vi "GetControlRefnumsOfTab__slk_mt.vi"(8 "error in (no error)":errorcluster, 11 "tab control refnum in":refnum<vi>) -> (0 "error out":errorcluster, 3 "control refnums out":refnum<vi>[](array[refnum]))   [LabVIEW 2010, in "Lazyboots Menu Tool.lvlib"]
doc: "Gets all control refnums from specified tab control."
uses:
  Library/Lazyboots Menu Tool.lvlib
panel:
  # "GetControlRefnumsOfTab__slk_mt.vi\nGets all control refnums from specified tab control.\n\nNOTICE -- YOU MUST LEAVE THIS NOTICE IN PLACE.\n\nCopyright (c) 2011, LIANG LIU Shawn.Liu.cn@gmail.com\nAll rights reserved.\n\nRedistribution and use in source and binary forms, with or without modification, are permitted provided that the following conditions are met:\n-Redistributions of source code must retain the above copyright notice, this list of conditions and the following disclaimer.\n-Redistributions in binary form must reproduce the above copyright notice, this list of conditions and the following disclaimer in the documentation and/or other materials provided with the distribution.\n-Neither the name of the eLp nor the names of its contributors may be used to endorse or promote products derived from this software without specific prior written permission.\n\nTHIS SOFTWARE IS PROVIDED BY THE COPYRIGHT HOLDERS AND CONTRIBUTORS \"AS IS\" AND ANY EXPRESS OR IMPLIED WARRANTIES, INCLUDING, BUT NOT LIMITED TO, THE IMPLIED WARRANTIES OF MERCHANTABILITY AND FITNESS FOR A PARTICULAR PURPOSE ARE DISCLAIMED. IN NO EVENT SHALL THE COPYRIGHT HOLDER OR CONTRIBUTORS BE LIABLE FOR ANY DIRECT, INDIRECT, INCIDENTAL, SPECIAL, EXEMPLARY, OR CONSEQUENTIAL DAMAGES (INCLUDING, BUT NOT LIMITED TO, PROCUREMENT OF SUBSTITUTE GOODS OR SERVICES; LOSS OF USE, DATA, OR PROFITS; OR BUSINESS INTERRUPTION) HOWEVER CAUSED AND ON ANY THEORY OF LIABILITY, WHETHER IN CONTRACT, STRICT LIABILITY, OR TORT (INCLUDING NEGLIGENCE OR OTHERWISE) ARISING IN ANY WAY OUT OF THE USE OF THIS SOFTWARE, EVEN IF ADVISED OF THE POSSIBILITY OF SUCH DAMAGE."
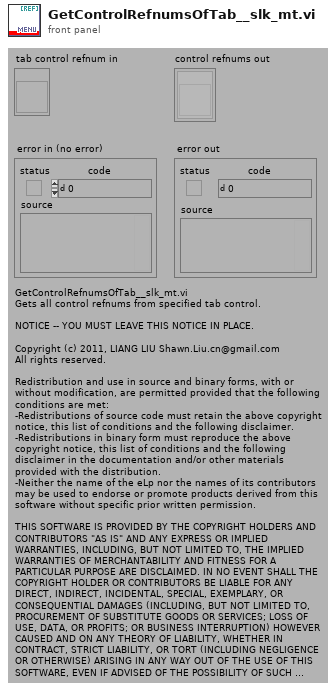
[diagram p1: front panel]
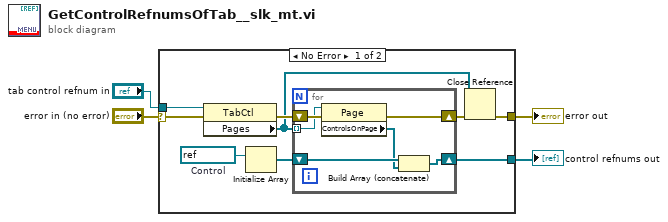
[diagram p0: block diagram]
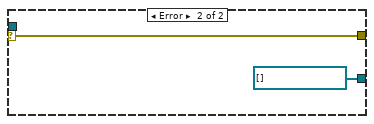
[diagram p2: hidden frame]
diagram:
  n1 = case shown="No Error" "error in (no error)" {
    selector: "error in (no error)" -> [w11 w21]
    tunnel: "tab control refnum in" -> [w13 _]
    tunnel: [w12 refnum<vi>[] []] -> w3
    tunnel: [w10 w21] -> w1
    frame No Error {
      w9 = refnum<vi> refnum  # Control
      n2 = property class="TabCtl"(reference=w13, error in=w11) -> (error out=w7:errorcluster, "Pages"=w5:refnum<vi>[])  [unwired: 1 out]
      n3 = Initialize Array(w9) -> (w8:refnum<vi>[])  [unwired: 1 in]
      n4 = for {
        tunnel: w5 -> [w18] mode=indexing
        shift-right: [w16] -> w12
        shift-left: w8 -> [w17]
        shift-right: [w15] -> w6
        shift-left: w7 -> [w19]
        n5 = property class="Page"(reference=w18, error in=w19) -> (error out=w15:errorcluster, "ControlsOnPage"=w14:refnum<vi>[])  [unwired: 1 out]
        n6 = Build Array (concatenate)(w17, w14) -> (w16:refnum<vi>[])
      }
      n7 = Close Reference(reference=w5, error in (no error)=w6) -> (error out=w10:errorcluster)
    }
    frame Error {
    }
  }
  "control refnums out" <- w3
  "error out" <- w1
